vi "New Station Config.vi"(9 "value":map{i32, T1}(c390), 10 "key":string, 11 "Station Config in":T2) -> (3 "Station Config out":T2)   [LabVIEW 2025, in "Full User Interface.lvlib"]
uses:
  Full User Interface.lvlib
  Station Config.ctl
  Station Info.ctl
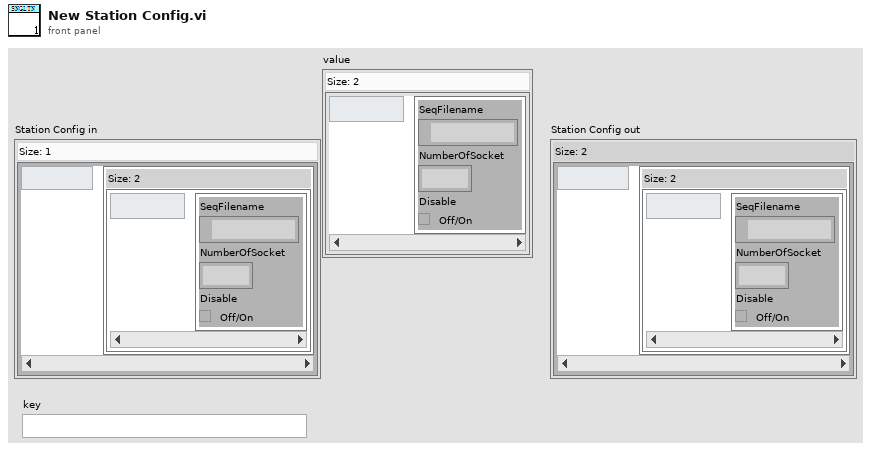
[diagram p1: front panel]
types:
  T1 = typedef "Full User Interface.lvlib/Station Info.ctl" = cluster{"SeqFilename":path, "NumberOfSocket":i32, "Disable":bool}
  T2 = typedef "Full User Interface.lvlib/Station Config.ctl" = map{string, map{i32, T1}}
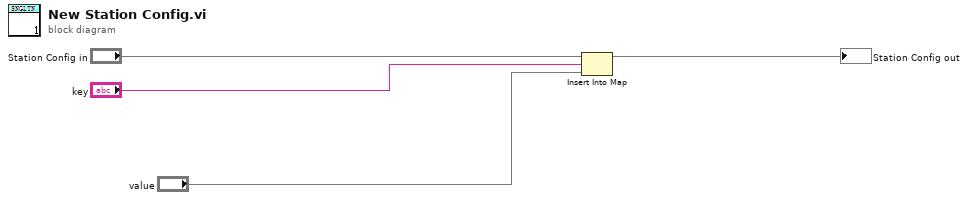
[diagram p0: block diagram]
diagram:
  n1 = Insert Into Map(map in="Station Config in", key="key", value="value") -> (map out=→"Station Config out":T2)  [unwired: 2 out]
